vi "UPS监控.vi"() -> ()   [LabVIEW 2016, in "环境动力监测库.lvlib"]
uses:
  <vilib>/Utility/miscctls.llb/LVPointTypeDef.ctl
  <vilib>/ptbypt/NI_PtbyPt.lvlib
panel:
  out "漏电报警累加值":u16 caption="漏电报警累加值："
  out "当前报警状态":u16(ring) caption="当前报警状态：" items=["无报警"=0, "过压报警"=1, "欠压报警"=2, "过流报警"=4, "漏电报警"=8]
  out "通讯状态":u16(ring) caption="通讯状态：" items=["正常", "异常"]
  out "过流报警累加值":u16 caption="过流报警累加值："
  out "欠压报警累加值":u16 caption="欠压报警累加值："
  out "过压报警累加值":u16 caption="过压报警累加值："
  out "当前漏电电流":dbl caption="当前漏电电流："
  out "当前电流":dbl caption="当前电流："
  out "当前电压":u16 caption="当前电压："
  # "UPS监测"
  # "mA"
  # "A"
  # "V"
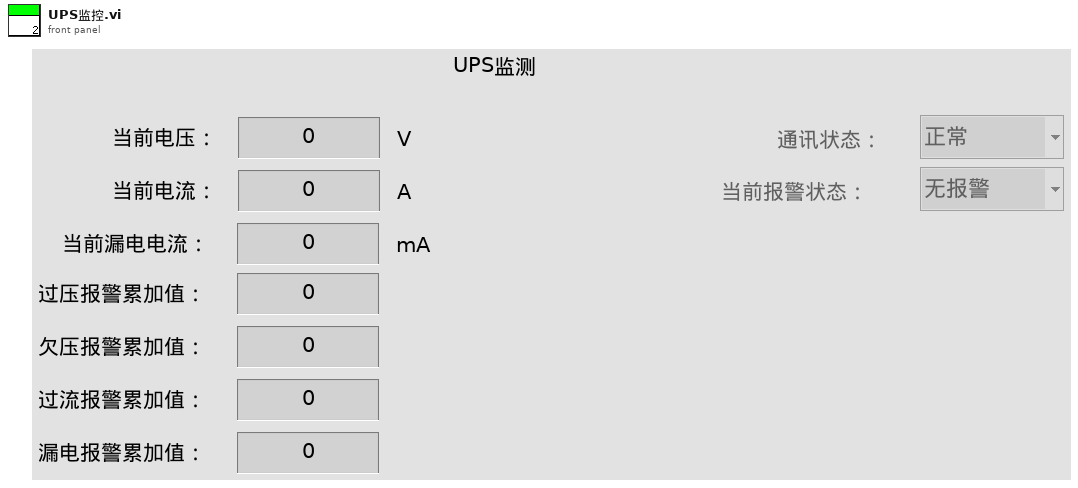
[diagram p1: front panel]
types:
  T1 = typedef "LVPointTypeDef.ctl" = cluster{"Horizontal":i16, "Vertical":i16}
  T2 = cluster{"时间标识":timestamp, "设备":string, "日志信息":string}
  T3 = cluster{"R0":i16, "R1":i16, "R2":i16, "R3":i16, "R4":i16, "R5":i16, "R6":i16, "R7":i16, "R8":i16, "R9":i16, "R10":i16, "R11":i16, "R12":i16, "R13":i16, "R14":i16, "R15":i16, "R16":i16, "R17":i16, "R18":i16, "R19":i16, "R20":i16, "R21":i16, "R22":i16, "R23":i16, "R24":i16, "R25":i16, "R26":i16, "R27":i16, "R28":i16, "R29":i16, "R30":i16, "R31":i16, "R32":i16, "R33":i16, "R34":i16, "R35":i16, "R36":i16, "R37":i16, "R38":i16, "R39":i16}
  T4 = cluster{"漏水监测输出":bool, "门禁监测输出":bool, "温湿度监测输出":bool, "烟雾监测输出":bool, "空调监测输出":bool, "自动重合闸输出":bool}
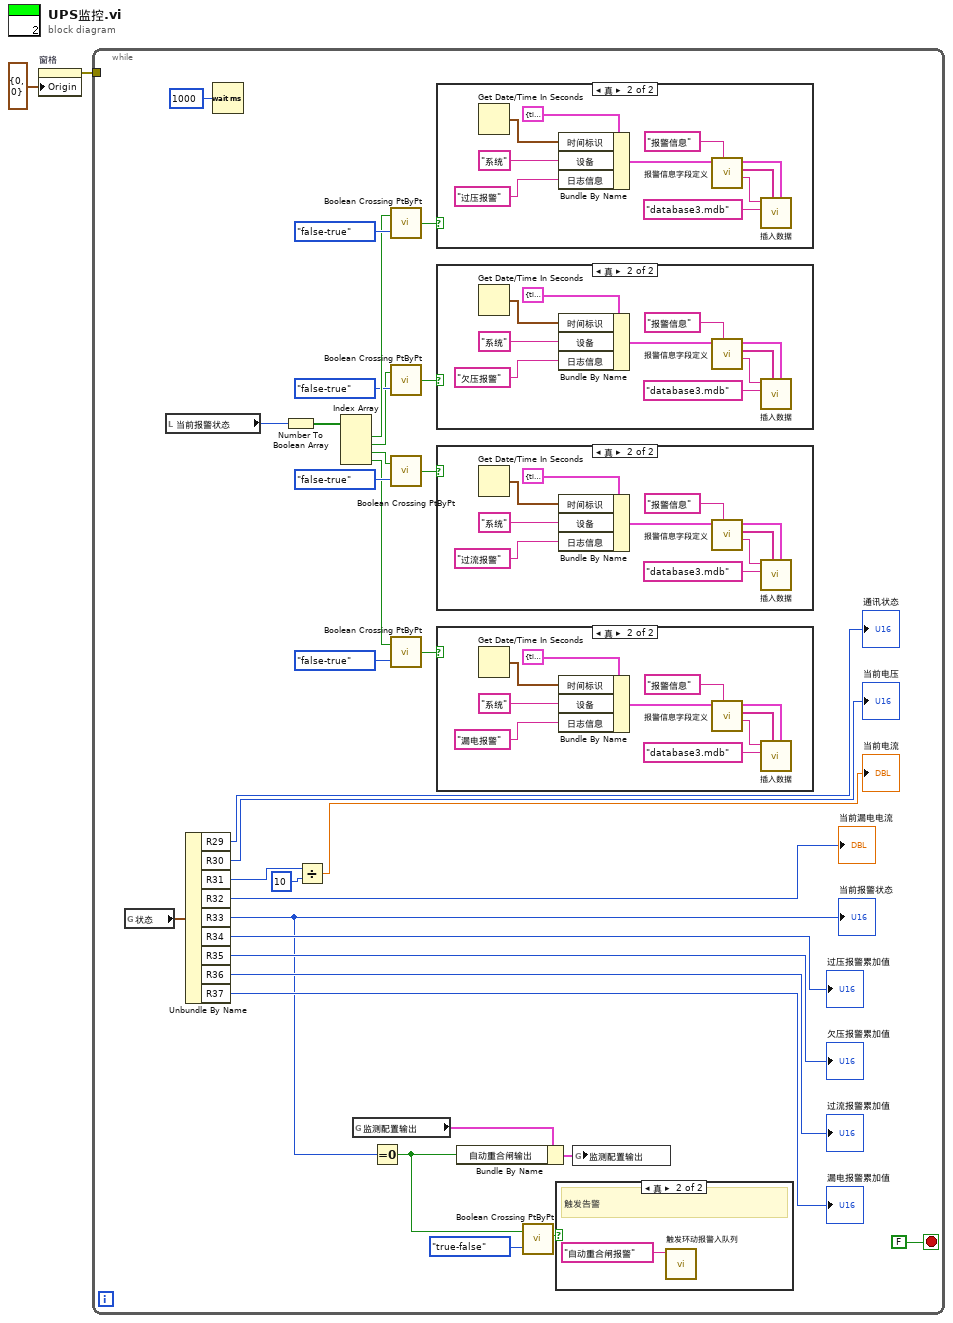
[diagram p0: block diagram]
diagram:
  n1 = property on="窗格" class="Pane"("Origin"=T1 {"Horizontal"=0, "Vertical"=0} ("原点")) -> (error out=w1:errorcluster)  [unwired: 2 in, 1 out]
  n2 = while {
    tunnel: w1 -> [_]
    stop <- FALSE stop-if-true
    n3 = global read "外部交互全局变量.vi" "状态"() -> (w25:T3)
    n4 = local read "当前报警状态"() -> (w24:u16)
    n5 = Unbundle By Name(w25) -> ("R29"=→"通讯状态":i16, "R30"=→"当前电压":i16, "R31"=w33:i16, "R32"=→"当前漏电电流":i16, "R33"=w6:i16, "R34"=→"过压报警累加值":i16, "R35"=→"欠压报警累加值":i16, "R36"=→"过流报警累加值":i16, "R37"=→"漏电报警累加值":i16)
    "当前报警状态" <- w6
    n6 = Wait (ms)(milliseconds to wait=u32 1000 ("等待时间（毫秒）")) -> ()  [unwired: 1 out]
    n7 = Number To Boolean Array(number=w24) -> (Boolean array=w23:bool[])
    n8 = Divide(x=w33, y=i16 10) -> (x/y=→"当前电流":dbl)
    n9 = Index Array(array=w23) -> (element #1=w21:bool, element #2=w15:bool, element #3=w14:bool, element #4=w11:bool)  [unwired: 4 in]
    n10 = global read "内部交互全局变量.vi" "监测配置输出"() -> (w8:T4)
    n11 = Equal To 0?(x=w6) -> (x = 0?=w3:bool)
    n12 = call <vilib>:"Boolean Crossing PtByPt.vi"("direction"=enum16{"either", "false-true", "true-false"}."false-true", "input"=w21) -> ("crossing"=w20:bool)  [unwired: 1 in]
    n13 = call <vilib>:"Boolean Crossing PtByPt.vi"("direction"=enum16{"either", "false-true", "true-false"}."false-true", "input"=w15) -> ("crossing"=w19:bool)  [unwired: 1 in]
    n14 = call <vilib>:"Boolean Crossing PtByPt.vi"("direction"=enum16{"either", "false-true", "true-false"}."false-true", "input"=w14) -> ("crossing"=w16:bool)  [unwired: 1 in]
    n15 = call <vilib>:"Boolean Crossing PtByPt.vi"("direction"=enum16{"either", "false-true", "true-false"}."false-true", "input"=w11) -> ("crossing"=w13:bool)  [unwired: 1 in]
    n16 = case shown="真" w20 {
      frame False {
      }
      frame True {
        n17 = Get Date/Time In Seconds() -> (seconds since 1Jan1904=w75:timestamp)
        n18 = Bundle By Name(cluster=T2 {"时间标识"=timestamp(0 s since 1904-01-01), "设备"="", "日志信息"=""} ("data in"), "时间标识"=w75, "设备"="系统", "日志信息"="过压报警") -> (w74:T2)
        n19 = call "报警信息字段定义.vi"("table输入"="报警信息", "data in"=w74) -> ("table输出"=w70:string, "columns"=w69:string[], "data out"=w68:T2)  [unwired: 7 in]
        n20 = call "插入数据.vi"("data"=w68, "columns"=w69, "database"="database3.mdb", "table"=w70) -> ()  [unwired: 7 in, 1 out]
      }
    }
    n21 = case shown="真" w19 {
      frame False {
      }
      frame True {
        n22 = Get Date/Time In Seconds() -> (seconds since 1Jan1904=w65:timestamp)
        n23 = Bundle By Name(cluster=T2 {"时间标识"=timestamp(0 s since 1904-01-01), "设备"="", "日志信息"=""} ("data in"), "时间标识"=w65, "设备"="系统", "日志信息"="欠压报警") -> (w64:T2)
        n24 = call "报警信息字段定义.vi"("table输入"="报警信息", "data in"=w64) -> ("table输出"=w60:string, "columns"=w59:string[], "data out"=w58:T2)  [unwired: 7 in]
        n25 = call "插入数据.vi"("data"=w58, "columns"=w59, "database"="database3.mdb", "table"=w60) -> ()  [unwired: 7 in, 1 out]
      }
    }
    n26 = case shown="真" w16 {
      frame False {
      }
      frame True {
        n27 = Get Date/Time In Seconds() -> (seconds since 1Jan1904=w55:timestamp)
        n28 = Bundle By Name(cluster=T2 {"时间标识"=timestamp(0 s since 1904-01-01), "设备"="", "日志信息"=""} ("data in"), "时间标识"=w55, "设备"="系统", "日志信息"="过流报警") -> (w54:T2)
        n29 = call "报警信息字段定义.vi"("table输入"="报警信息", "data in"=w54) -> ("table输出"=w50:string, "columns"=w49:string[], "data out"=w48:T2)  [unwired: 7 in]
        n30 = call "插入数据.vi"("data"=w48, "columns"=w49, "database"="database3.mdb", "table"=w50) -> ()  [unwired: 7 in, 1 out]
      }
    }
    n31 = case shown="真" w13 {
      frame False {
      }
      frame True {
        n32 = Get Date/Time In Seconds() -> (seconds since 1Jan1904=w45:timestamp)
        n33 = Bundle By Name(cluster=T2 {"时间标识"=timestamp(0 s since 1904-01-01), "设备"="", "日志信息"=""} ("data in"), "时间标识"=w45, "设备"="系统", "日志信息"="漏电报警") -> (w44:T2)
        n34 = call "报警信息字段定义.vi"("table输入"="报警信息", "data in"=w44) -> ("table输出"=w40:string, "columns"=w39:string[], "data out"=w38:T2)  [unwired: 7 in]
        n35 = call "插入数据.vi"("data"=w38, "columns"=w39, "database"="database3.mdb", "table"=w40) -> ()  [unwired: 7 in, 1 out]
      }
    }
    n36 = Bundle By Name(cluster=w8, "自动重合闸输出"=w3) -> (w7:T4)
    n37 = call <vilib>:"Boolean Crossing PtByPt.vi"("direction"=enum16{"either", "false-true", "true-false"}."true-false", "input"=w3) -> ("crossing"=w4:bool)  [unwired: 1 in]
    n38 = case shown="真" w4 {
      frame False {
      }
      frame True {
        # "触发告警"
        n39 = call "触发环动报警入队列.vi"("报警内容"="自动重合闸报警") -> ()  [unwired: 11 in]
      }
    }
    n40 = global write "内部交互全局变量.vi" "监测配置输出"(w7) -> ()
  }
